vi "Crosstalk (N Chan).vi"(0 "stimulus signal":waveform(dbl), 1 "idle channel response":waveform(dbl)[](array[waveform]), 3 "advanced span [Hz]":dbl=-1.0 format="%.2f", 5 "error in (no error)":errorcluster, 6 "desired units":T10, 9 "expected fundamental frequency [Hz]":dbl=-1.0 format="%.2f") -> (11 "detected tone idle-channel response":cluster{"frequency [Hz]":dbl, "amplitude":dbl}[](array[cluster]), 12 "unit labels":T9, 13 "detected tone stimulus":cluster{"frequency [Hz]":dbl, "amplitude":dbl}={"frequency [Hz]"=nan, "amplitude"=nan} {"amplitude" format="%.3f"; "frequency [Hz]" format="%.2f"}, 14 "complex spectrum\nstimulus X":T8={"complex spectrum response"={"f0"=0.0, "df"=1.0, "complex spectrum"=[]}, "spectrum info"={"channel name"="", "description"="", "x-axis units"=0, "spectral info"={"spectrum type"=enum."Power [Magnitude^2]", "linear/dB"=enum."linear", "window"=0, "window size"=0, "FFT size"=0}, "engineering units"=0, "custom label"="", "dB reference [EU]"=0.0, "peak units"=enum."rms", "weighting filter"=0, "spectral density?"=FALSE, "unit label"="", "spectrum skewed?"=FALSE, "complimentary spectrum units"=enum."none"}} {"spectrum info"."x-axis units" items=["Time (s)"=0, "Frequency-CB (Hz)"=1, "Frequency-CPB (Hz)"=1248, "Frequency-Arbitrary (Hz)"=2357, "Quefrency (s)"=2, "Revolutions (rev)"=3, "Order"=4, "Speed (RPM)"=11, "Speed (rad/s)"=21, "Index"=65535]; "spectrum info"."weighting filter" items=["Linear", "A-weighting", "B-weighting", "C-weighting", "ITU-R 468-4", "Dolby", "CCITT", "C-message", "Wb", "Wc", "Wd", "We", "Wf", "Wh", "Wj", "Wk", "Wm", "AES17 20 kHz lowpass", "AES17 40 kHz lowpass", "AES17 20 kHz highpass", "AES17 40 kHz highpass"]; "spectrum info"."dB reference [EU]" format="%.2f"; "spectrum info"."engineering units" items=["custom..."=0, "V"=1, "A"=21, "C"=30, "pC"=31, "s"=32, "-"=29, "Pa"=2, "N"=20, "g"=3, "m/s^2"=4, "m/s"=5, "m"=6, "mm/s"=12, "mm"=13, "micron/s"=14, "micron"=15, "in/s^2"=7, "in/s"=8, "in"=9, "mil/s"=10, "mil"=11, "rad/s^2"=16, "rad/s"=17, "rad"=18, "deg/s^2"=26, "deg/s"=27, "deg"=28, "RPM"=22, "cycle/s^2"=23, "Hz"=24, "cycle"=25, "strain"=19]; "spectrum info"."spectral info"."window" items=["None "=0, "Hanning"=1, "Hamming"=2, "Blackman-Harris"=3, "Exact Blackman"=4, "Blackman"=5, "Flat Top"=6, "4 Term B-Harris "=7, "7 Term B-Harris"=8, "Low Sidelobe"=9, "Force - Exponential"=10, "Gaussian"=62]; "complex spectrum response"."complex spectrum" format="%.2f"; "complex spectrum response"."df" format="%.2f"; "complex spectrum response"."f0" format="%.2f"}, 15 "complex spectrum idle-channel response":T7(array[cluster]) {"spectrum info"."x-axis units" items=["Time (s)"=0, "Frequency-CB (Hz)"=1, "Frequency-CPB (Hz)"=1248, "Frequency-Arbitrary (Hz)"=2357, "Quefrency (s)"=2, "Revolutions (rev)"=3, "Order"=4, "Speed (RPM)"=11, "Speed (rad/s)"=21, "Index"=65535]; "spectrum info"."weighting filter" items=["Linear", "A-weighting", "B-weighting", "C-weighting", "ITU-R 468-4", "Dolby", "CCITT", "C-message", "Wb", "Wc", "Wd", "We", "Wf", "Wh", "Wj", "Wk", "Wm", "AES17 20 kHz lowpass", "AES17 40 kHz lowpass", "AES17 20 kHz highpass", "AES17 40 kHz highpass"]; "spectrum info"."dB reference [EU]" format="%.2f"; "spectrum info"."engineering units" items=["custom..."=0, "V"=1, "A"=21, "C"=30, "pC"=31, "s"=32, "-"=29, "Pa"=2, "N"=20, "g"=3, "m/s^2"=4, "m/s"=5, "m"=6, "mm/s"=12, "mm"=13, "micron/s"=14, "micron"=15, "in/s^2"=7, "in/s"=8, "in"=9, "mil/s"=10, "mil"=11, "rad/s^2"=16, "rad/s"=17, "rad"=18, "deg/s^2"=26, "deg/s"=27, "deg"=28, "RPM"=22, "cycle/s^2"=23, "Hz"=24, "cycle"=25, "strain"=19]; "spectrum info"."spectral info"."window" items=["None "=0, "Hanning"=1, "Hamming"=2, "Blackman-Harris"=3, "Exact Blackman"=4, "Blackman"=5, "Flat Top"=6, "4 Term B-Harris "=7, "7 Term B-Harris"=8, "Low Sidelobe"=9, "Force - Exponential"=10, "Gaussian"=62]}, 16 "crosstalk":dbl[](array[numeric]), 17 "phase lag":dbl[](array[numeric]), 19 "error out":errorcluster)   [LabVIEW 2023]
uses:
  <vilib>/addons/_NISVFA/_Shared subVIs/Controls/svc_Spectrum Info.ctl
  <vilib>/addons/_NISVFA/_Shared subVIs/Controls/svc_X-Axis Units.ctl
  <vilib>/addons/_NISVFA/_Shared subVIs/Controls/svc_Spectrum Type.ctl
  <vilib>/addons/_NISVFA/_Shared subVIs/Controls/svc_Engineering Units Text Ring.ctl
  <vilib>/addons/_NISVFA/_Shared subVIs/Controls/svc_Weighting Filter Text Ring.ctl
  <vilib>/addons/_NISVFA/_Shared subVIs/Controls/svc_Complimentary Spectrum Units.ctl
  <vilib>/addons/_NISVFA/_Shared subVIs/Controls/svc_Window.ctl
  <vilib>/addons/Sound and Vibration/svt_Distortion/SoundVib_Distortion.lvlib
  <vilib>/addons/Sound and Vibration/svt_Single Tone Measurements/SoundVib_SingleTone.lvlib
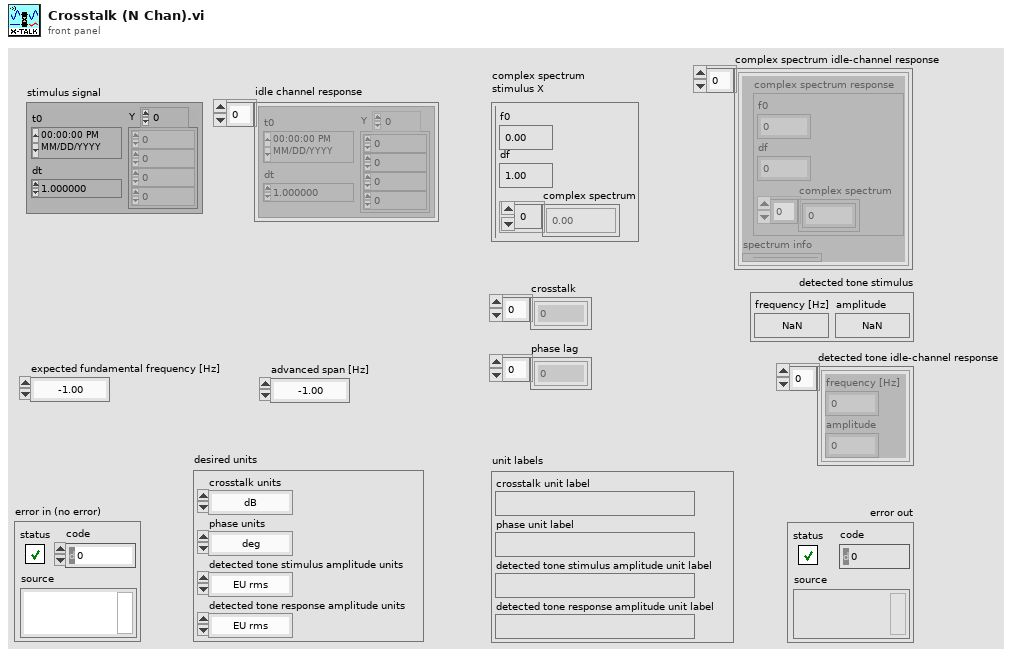
[diagram p1: front panel]
types:
  T1 = typedef "svc_Spectrum Info.ctl" = cluster{"channel name":string, "description":string, "x-axis units":T2, "spectral info":cluster{"spectrum type":T3, "linear/dB":enum16{"linear", "dB"}, "window":u16, "window size":i32, "FFT size":i32}, "engineering units":T4, "custom label":string, "dB reference [EU]":dbl, "peak units":enum16{"rms", "peak", "peak-peak"}, "weighting filter":T5, "spectral density?":bool, "unit label":string, "spectrum skewed?":bool, "complimentary spectrum units":T6}
  T2 = typedef "svc_X-Axis Units.ctl" = u16
  T3 = typedef "svc_Spectrum Type.ctl" = enum16{"FFT Spectrum [complex]", "Amplitude [Magnitude]", "Power [Magnitude^2]", "Cross Spectrum [complex]", "Frequency Response [Complex]"}
  T4 = typedef "svc_Engineering Units Text Ring.ctl" = u16
  T5 = typedef "svc_Weighting Filter Text Ring.ctl" = u16
  T6 = typedef "svc_Complimentary Spectrum Units.ctl" = enum16{"none", "radians", "degrees", "cycles", "imaginary"}
  T7 = cluster{"complex spectrum response":cluster{"f0":dbl, "df":dbl, "complex spectrum":cdb[]}, "spectrum info":T1}[]
  T8 = cluster{"complex spectrum response":cluster{"f0":dbl, "df":dbl, "complex spectrum":cdb[]}, "spectrum info":T1}
  T9 = cluster{"crosstalk unit label":string, "phase unit label":string, "detected tone stimulus amplitude unit label":string, "detected tone response amplitude unit label":string}
  T10 = cluster{"crosstalk units":enum16{"dB", "linear ratio"}, "phase units":enum16{"deg", "rad"}, "detected tone stimulus amplitude units":enum16{"EU rms", "EU peak", "EU peak-peak"}, "detected tone response amplitude units":enum16{"EU rms", "EU peak", "EU peak-peak"}}
  T11 = cluster{"crosstalk unit label":string, "phase unit label":string, "detected tone stimulus unit label":string, "detected response stimulus unit label":string}
  T12 = typedef "svc_Window.ctl" = u32
  T13 = cluster{"complex spectrum":cluster{"f0":dbl, "df":dbl, "complex spectrum":cdb[]}, "spectrum info":T1}
  T14 = cluster{"complex spectrum":cluster{"f0":dbl, "df":dbl, "complex spectrum":cdb[]}, "spectrum info":T1}[]
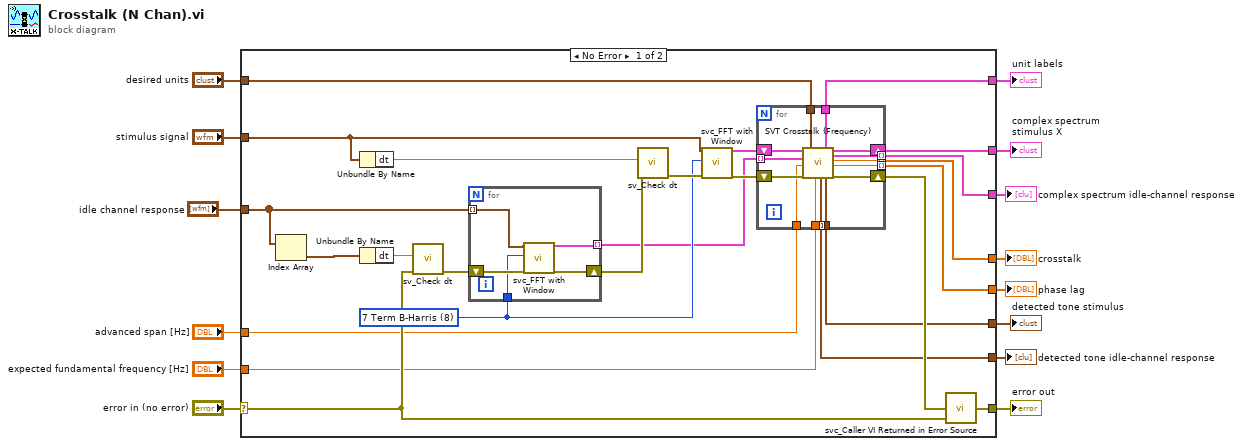
[diagram p0: block diagram]
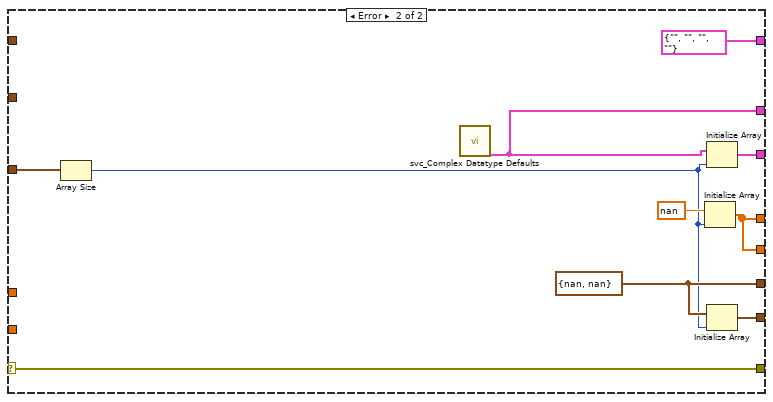
[diagram p2: hidden frame]
diagram:
  n1 = case shown="No Error" "error in (no error)" {
    selector: "error in (no error)" -> [w20 w68]
    tunnel: "idle channel response" -> [w16 w66]
    tunnel: "stimulus signal" -> [w21 _]
    tunnel: [w31 w68] -> w13
    tunnel: [w38 w62] -> w2
    tunnel: "desired units" -> [w37 _]
    tunnel: [w36 T11 {"crosstalk unit label"="", "phase unit label"="", "detected tone stimulus unit label"="", "detected response stimulus unit label"=""} ("unit labels")] -> w10
    tunnel: [w28 w64] -> w3
    tunnel: [w34 w61] -> w9
    tunnel: [w33 w59] -> w4
    tunnel: [w32 w62] -> w1
    tunnel: [w29 w65] -> w8
    tunnel: "expected fundamental frequency [Hz]" -> [w19 _]
    tunnel: "advanced span [Hz]" -> [w18 _]
    frame No Error {
      w24 = T12 8 items=["None ", "Hanning", "Hamming", "Blackman-Harris", "Exact Blackman", "Blackman", "Flat Top", "4 Term B-Harris ", "7 Term B-Harris", "Low Sidelobe"] ("window")
      n2 = Index Array(array=w16) -> (element=w17:waveform(dbl))  [unwired: 1 in]
      n3 = Unbundle By Name(w21) -> ("dt"=w23:dbl)
      n4 = Unbundle By Name(w17) -> ("dt"=w22:dbl)
      n5 = call <vilib>:"sv_Check dt.vi"("error in"=w20, "dt"=w22) -> ("error out"=w27:errorcluster)  [unwired: 8 in, 1 out]
      n6 = for {
        tunnel: w24 -> [w56]
        shift-right: [w57] -> w26
        shift-left: w27 -> [w58]
        tunnel: w16 -> [w55] mode=indexing
        tunnel: [w54] -> w15 mode=indexing
        n7 = call <vilib>:"svc_FFT with Window.vi"("time signal in [EU]"=w55, "window"=w56, "error in"=w58) -> ("complex spectrum"=w54:T8, "error out"=w57:errorcluster)  [unwired: 15 in]
      }
      n8 = call <vilib>:"sv_Check dt.vi"("error in"=w26, "dt"=w23) -> ("error out"=w25:errorcluster)  [unwired: 8 in, 1 out]
      n9 = call <vilib>:"svc_FFT with Window.vi"("time signal in [EU]"=w21, "window"=w24, "error in"=w25) -> ("complex spectrum"=w35:T8, "error out"=w30:errorcluster)  [unwired: 15 in]
      n10 = for {
        tunnel: [w52] -> w38 mode=indexing
        tunnel: w37 -> [w51]
        tunnel: [w50] -> w36
        tunnel: [w48] -> w34
        tunnel: [w47] -> w33 mode=indexing
        tunnel: [w46] -> w32 mode=indexing
        tunnel: [w43] -> w28 mode=indexing
        tunnel: w19 -> [w42]
        tunnel: w18 -> [w41]
        shift-right: [w44] -> w29
        shift-left: w35 -> [w49]
        shift-right: [w53] -> w39
        shift-left: w30 -> [w45]
        tunnel: w15 -> [w40] mode=indexing
        n11 = call <vilib>:"SVT Crosstalk (Frequency).vi"("complex spectrum\nstimulus X"=w49, "complex spectrum\nidle-channel response Y"=w40, "advanced span [Hz]"=w41, "error in (no error)"=w45, "desired units"=w51, "expected fundamental frequency [Hz]"=w42) -> ("detected tone idle-channel response"=w47:cluster{"frequency [Hz]":dbl, "amplitude":dbl}, "unit labels"=w50:T9, "detected tone stimulus"=w48:cluster{"frequency [Hz]":dbl, "amplitude":dbl}, "dup complex spectrum\nstimulus X"=w44:T8, "dup complex spectrum\nidle-channel response Y"=w43:T8, "crosstalk"=w52:dbl, "phase lag"=w46:dbl, "error out"=w53:errorcluster)  [unwired: 6 in]
      }
      n12 = call <vilib>:"svc_Caller VI Returned in Error Source.vi"("warning input to caller"=w20, "error in"=w39) -> ("error out"=w31:errorcluster)  [unwired: 3 in]
    }
    frame Error {
      w61 = cluster{"frequency [Hz]":dbl, "amplitude":dbl} {"frequency [Hz]"=nan, "amplitude"=nan} ("detected tone stimulus")
      n13 = Array Size(array=w66) -> (size(s)=w60:i32)
      n14 = call <vilib>:"svc_Complex Datatype Defaults.vi"() -> ("complex spectrum"=w65:T13)  [unwired: 11 in, 8 out]
      n15 = Initialize Array(nan ("phase lag"), w60) -> (w62:dbl[])
      n16 = Initialize Array(w65, w60) -> (w64:T14)
      n17 = Initialize Array(w61, w60) -> (w59:cluster{"frequency [Hz]":dbl, "amplitude":dbl}[])
    }
  }
  "error out" <- w13
  "unit labels" <- w10
  "complex spectrum\nstimulus X" <- w8
  "detected tone stimulus" <- w9
  "detected tone idle-channel response" <- w4
  "complex spectrum idle-channel response" <- w3
  "crosstalk" <- w2
  "phase lag" <- w1
